vi "探头数据读取.vi"(11 "编号":string) -> ()   [LabVIEW 2016, in "斯坦道多参数.lvlib"]
panel:
  out "运行状态":u16(ring) items=["空闲", "水样测试", "标样核查"]
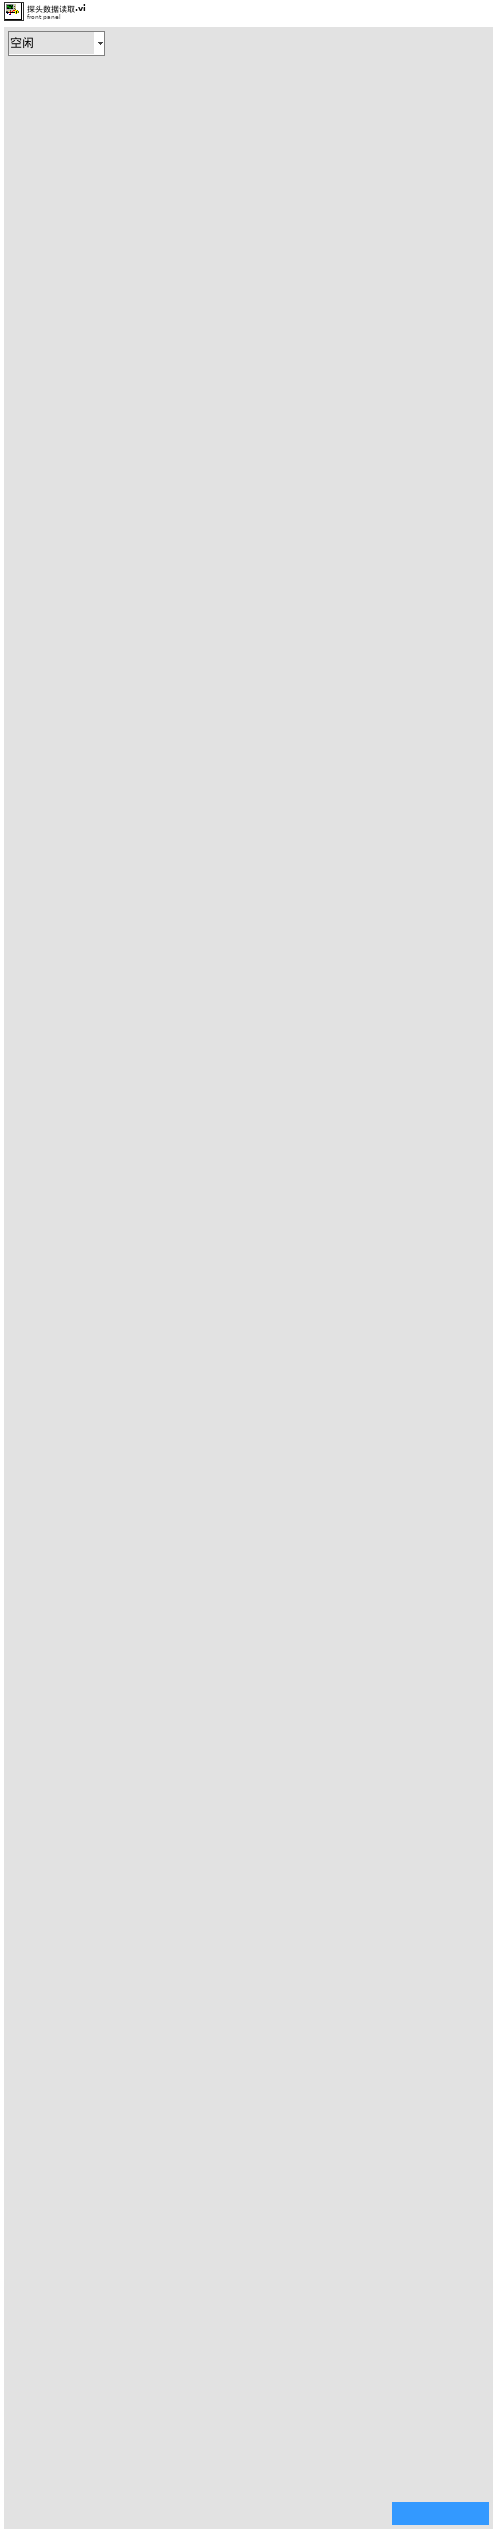
[diagram p1: front panel]
types:
  T1 = enum16{"pH", "DO", "Cond", "Turb", "ORP", "叶绿素a", "藻密度"}
  T2 = cluster{"温度测量值":sgl, "测量值":sgl, "温度偏移修正值":sgl, "信号值":sgl}
  T3 = cluster{"温度测量值":sgl, "DO%":sgl, "DOmg/L":sgl, "温度偏移修正值":sgl}
  T4 = cluster{"CH":u16, "监测值":dbl, "温度偏移修正值":sgl, "信号值":sgl}
  T5 = cluster{"pH探头选择":u16, "DO探头选择":u16, "电导率探头选择":u16, "浊度探头选择":u16, "叶绿素a探头选择":u16, "蓝绿藻探头选择":u16, "orp探头选择":u16}
  T6 = cluster{"电极状态标志":u16, "电极型号标志":u16, "酸碱度测量值":sgl, "温度测量值":sgl, "酸碱度信号值":sgl, "温度信号值":sgl, "酸碱度偏移修正值":sgl, "温度偏移修正值":sgl, "手动温度补偿值":sgl, "酸碱度电极零点":sgl, "酸碱度电极斜率":sgl, "第1点标准值记录":sgl, "第1点信号值记录":sgl, "第1点温度值记录":sgl, "第2点标准值记录":sgl, "第2点信号值记录":sgl, "第2点温度值记录":sgl, "命令滤波设定":u16, "温度模式":enum16{"ATC", "MTC"}, "生产批次":u16, "电极序号":u16, "串口地址":u16, "串口波特率":enum16{"9600", "19200", "115200"}, "串口校验位":enum16{"NONE", "ODD", "EVEN"}, "串口停止位":enum16{"1bit", "2bit"}, "第一点标准值":sgl, "第二点标准值":sgl}
  T7 = cluster{"报警码":u16, "pH数值":sgl, "0X0003_NC":sgl, "温度数据":sgl, "pH原始信号 mv":sgl, "0X0009_NC":string, "产品名称":string, "序列号":string, "硬件版本":string, "软件版本":string, "通讯地址":u16, "波特率":u16, "设备类型":u16, "0X0026_NC":string, "第一点原始数据":sgl, "第一点校准数据":sgl, "第二点原始数据":sgl, "第二点校准数据":sgl, "探头校准命令":u16, "温度校准参数":sgl, "温度校准命令":u16}
  T8 = cluster{"电极状态标志":u16, "电极型号标志":u16, "电导率测量值":sgl, "温度测量值":sgl, "电导率信号值":sgl, "温度信号值":sgl, "温度补偿系数":sgl, "电导率偏移修正值":sgl, "温度偏移修正值":sgl, "手动温度补偿值":sgl, "电导率电极零点":sgl, "电导率电极斜率":sgl, "命令滤波设定":u16, "温度模式":enum16{"ATC", "MTC"}, "生产批次":u16, "电极序号":u16, "串口地址":u16, "串口波特率":enum16{"9600", "19200", "115200"}, "串口校验位":enum16{"NONE", "ODD", "EVEN"}, "串口停止位":enum16{"1bit", "2bit"}, "第一点标准值":sgl, "第二点标准值":sgl}
  T9 = cluster{"报警码":u16, "电导率数据（uS/cm）":sgl, "0x0003 NC":sgl, "温度数据":sgl, "电导率原始信号电阻":sgl, "当前量程":u16, "温度补偿系数":sgl, "0X0009_NC":string, "产品名称":string, "序列号":string, "硬件版本":string, "软件版本":string, "通讯地址":u16, "波特率":u16, "设备类型":u16, "0X0026_NC":string, "第一点原始数据":sgl, "第一点校准数据":sgl, "0X0035_NC":sgl, "0X0037_NC":sgl, "探头校准命令":u16, "温度校准参数":sgl, "温度校准命令":u16}
  T10 = cluster{"电极状态标志":u16, "电极型号标志":u16, "溶解氧测量值":sgl, "温度测量值":sgl, "溶解氧饱和度值":sgl, "盐度补偿值":sgl, "大气压补偿值":sgl, "溶解氧偏移修正值":sgl, "温度偏移修正值":sgl, "手动温度补偿值":sgl, "溶解氧电极零点":sgl, "溶解氧电极斜率":sgl, "第1点标准值记录":sgl, "第1点信号值记录":sgl, "第1点温度值记录":sgl, "第2点标准值记录":sgl, "第2点信号值记录":sgl, "第2点温度值记录":sgl, "命令滤波设定":u16, "温度模式":enum16{"ATC", "MTC"}, "生产批次":u16, "电极序号":u16, "串口地址":u16, "串口波特率":enum16{"9600", "19200", "115200"}, "串口校验位":enum16{"NONE", "ODD", "EVEN"}, "串口停止位":enum16{"1bit", "2bit"}, "第一点标准值":sgl, "第二点标准值":sgl}
  T11 = cluster{"报警码":u16, "溶解氧数值（mg/L）":sgl, "溶解氧数据（%）":sgl, "温度数据":sgl, "溶解氧原始信号 nA":sgl, "大气压力":sgl, "盐度":sgl, "0X0009_NC":string, "产品名称":string, "序列号":string, "硬件版本":string, "软件版本":string, "通讯地址":u16, "波特率":u16, "设备类型":u16, "0X0026_NC":string, "第一点原始数据":sgl, "0X0033 NC":sgl, "第二点原始数据":sgl, "0X0037 NC":sgl, "探头校准命令":u16, "温度校准参数":sgl, "温度校准命令":u16}
  T12 = cluster{"电极状态标志":u16, "电极型号标志":u16, "浊度测量值":sgl, "温度测量值":sgl, "浊度信号值":sgl, "浊度偏移修正值":sgl, "温度偏移修正值":sgl, "手动温度补偿值":sgl, "浊度电极零点":sgl, "浊度电极斜率":sgl, "第1点标准值记录":sgl, "第1点信号值记录":sgl, "第1点温度值记录":sgl, "第2点标准值记录":sgl, "第2点信号值记录":sgl, "第2点温度值记录":sgl, "命令滤波设定":u16, "温度模式":enum16{"ATC", "MTC"}, "生产批次":u16, "电极序号":u16, "串口地址":u16, "串口波特率":enum16{"9600", "19200", "115200"}, "串口校验位":enum16{"NONE", "ODD", "EVEN"}, "串口停止位":enum16{"1bit", "2bit"}, "第一点标准值":sgl, "第二点标准值":sgl, "第三点标准值":sgl}
  T13 = cluster{"报警码":u16, "浊度数值 NTU":sgl, "温度数据":sgl, "原始光强数值":u16, "量程":u16, "平均次数":u16, "清扫模式":u16, "清扫次数":u16, "清扫间隔分钟":u16, "0X000B_NC":string, "产品名称":string, "序列号":string, "硬件版本":string, "软件版本":string, "通讯地址":u16, "波特率":u16, "设备类型":u16, "0X0026_NC":string, "校准量程":u16, "第一点原始光强":u16, "第一点校准数据":sgl, "第二点原始光强":u16, "第二点校准数据":sgl, "第三点原始光强":u16, "第三点校准数据":sgl, "探头校准命令":u16, "温度校准参数":sgl, "温度校准命令":u16}
  T14 = cluster{"电极状态标志":u16, "电极型号标志":u16, "测量值":sgl, "温度测量值":sgl, "信号值":sgl, "温度信号值":sgl, "000AH_NC":sgl, "偏移修正值":sgl, "温度偏移修正值":sgl, "手动温度补偿值":sgl, "命令滤波设定":u16, "温度模式":enum16{"ATC", "MTC"}, "生产批次":u16, "传感器序号":u16, "串口地址":u16, "串口波特率":enum16{"9600", "19200", "115200"}, "串口校验位":enum16{"NONE", "ODD", "EVEN"}, "串口停止位":enum16{"1bit", "2bit"}}
  T15 = cluster{"报警码":u16, "叶绿素a":sgl, "温度数据":sgl, "原始光强数值":u16, "量程":u16, "平均次数":u16, "清扫模式":u16, "清扫次数":u16, "清扫间隔分钟":u16, "0X000B_NC":string, "产品名称":string, "序列号":string, "硬件版本":string, "软件版本":string, "通讯地址":u16, "波特率":u16, "设备类型":u16, "0X0026_NC":string, "校准量程":u16, "第一点原始光强":u16, "第一点校准数据":sgl, "第二点原始光强":u16, "第二点校准数据":sgl, "第三点原始光强":u16, "第三点校准数据":sgl, "探头校准命令":u16, "温度校准参数":sgl, "温度校准命令":u16}
  T16 = cluster{"报警码":u16, "蓝绿藻":sgl, "温度数据":sgl, "原始光强数值":u16, "0X0006_NC":u16, "平均次数":u16, "清扫模式":u16, "清扫次数":u16, "清扫间隔分钟":u16, "0X000B_NC":string, "产品名称":string, "序列号":string, "硬件版本":string, "软件版本":string, "通讯地址":u16, "波特率":u16, "设备类型":u16, "0X0026_NC":string, "0X0030_NC":u16, "第一点原始光强":u16, "第一点校准数据":sgl, "第二点原始光强":u16, "第二点校准数据":sgl, "第三点原始光强":u16, "第三点校准数据":sgl, "探头校准命令":u16, "温度校准参数":sgl, "温度校准命令":u16}
  T17 = enum16{"pH", "DO", "Cond", "Turb", "ORP", "叶绿素a", "藻密度"}[]
  T18 = cluster{"ph":bool, "DO":bool, "Cond":bool, "Turb":bool, "叶绿素a":bool, "藻密度":bool, "ORP":bool}
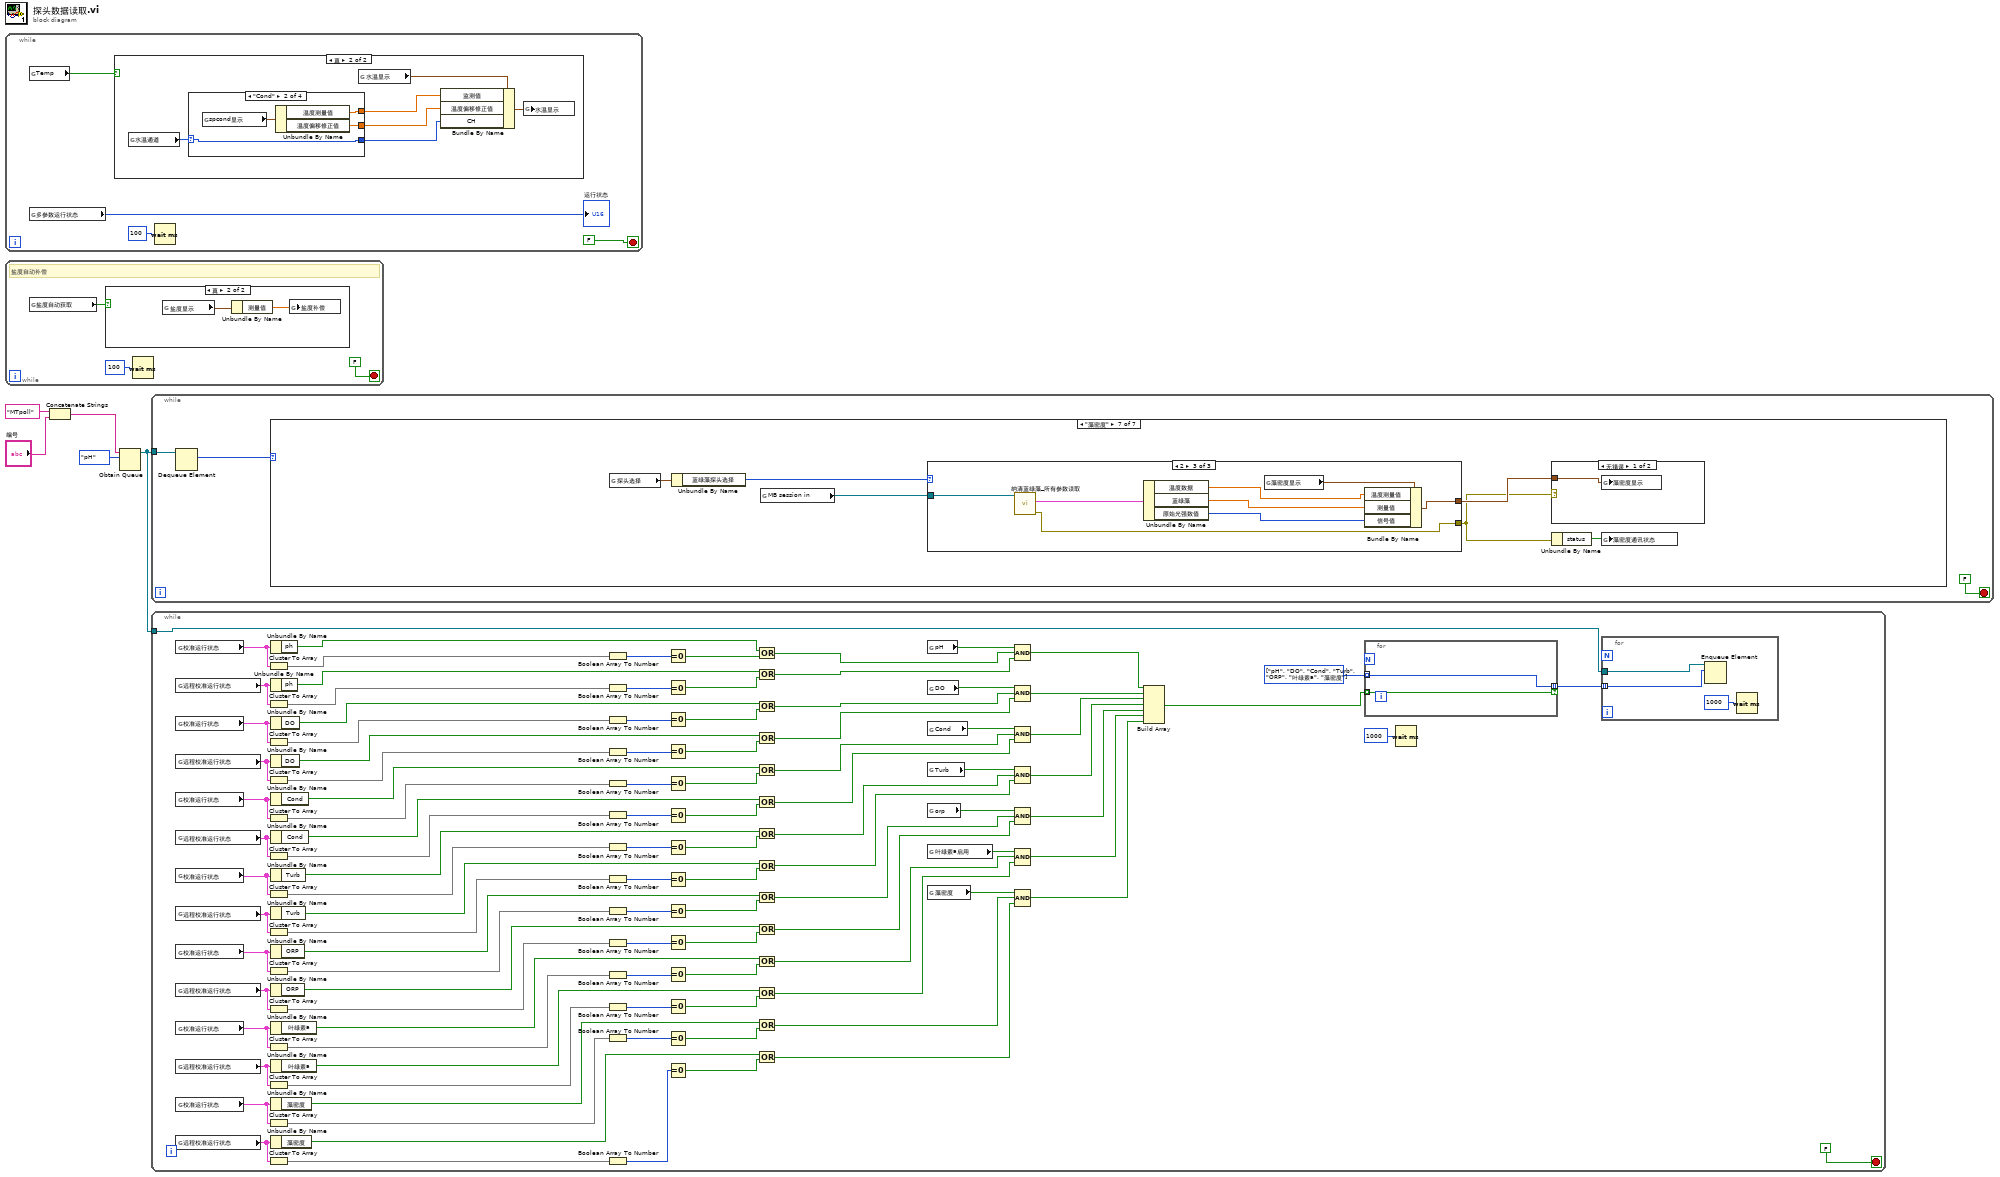
[diagram p0: block diagram]
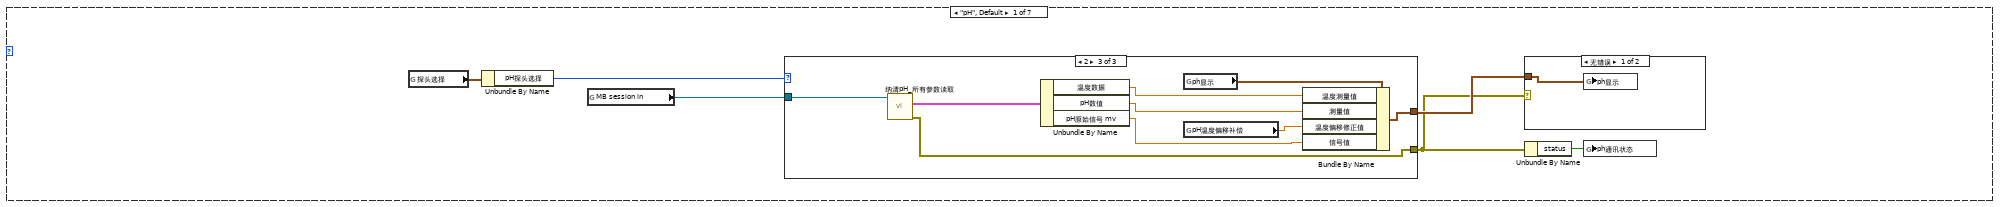
[diagram p2: hidden frame]
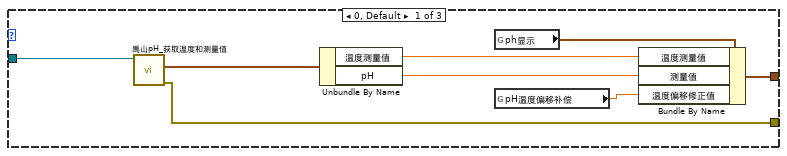
[diagram p3: hidden frame]
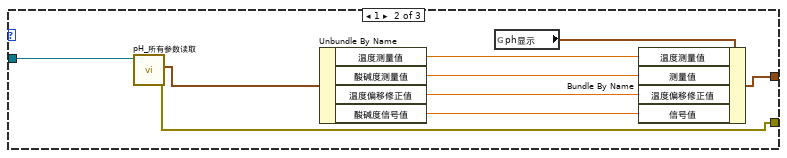
[diagram p4: hidden frame]
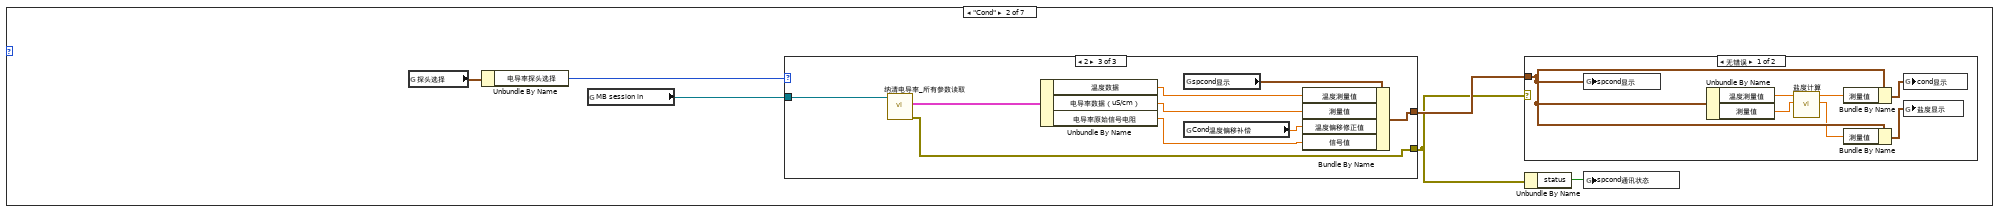
[diagram p6: hidden frame]
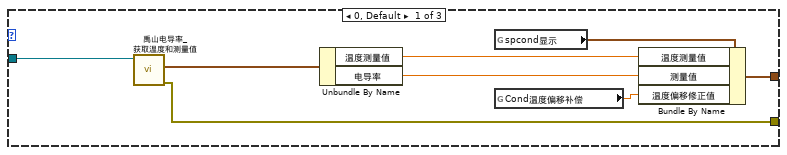
[diagram p7: hidden frame]
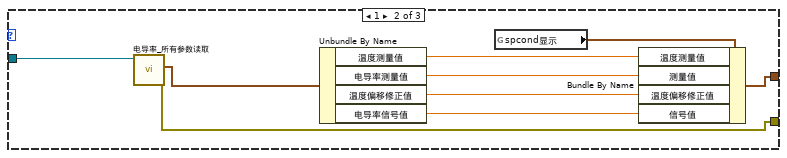
[diagram p8: hidden frame]
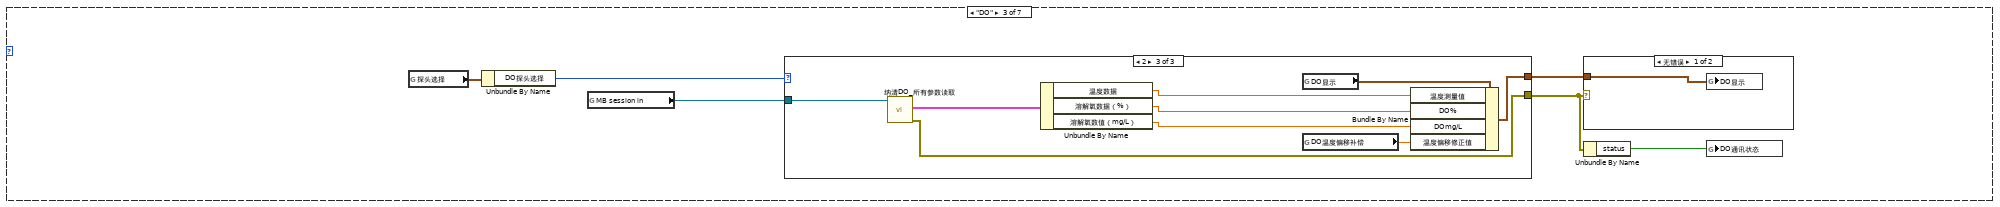
[diagram p10: hidden frame]
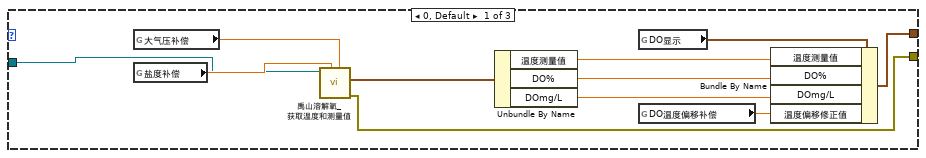
[diagram p11: hidden frame]
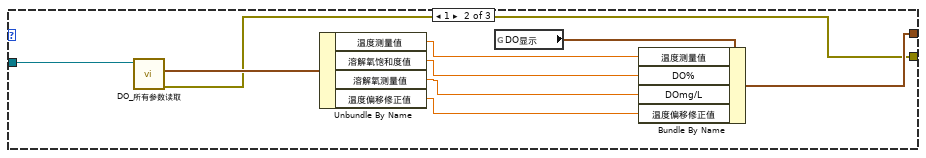
[diagram p12: hidden frame]
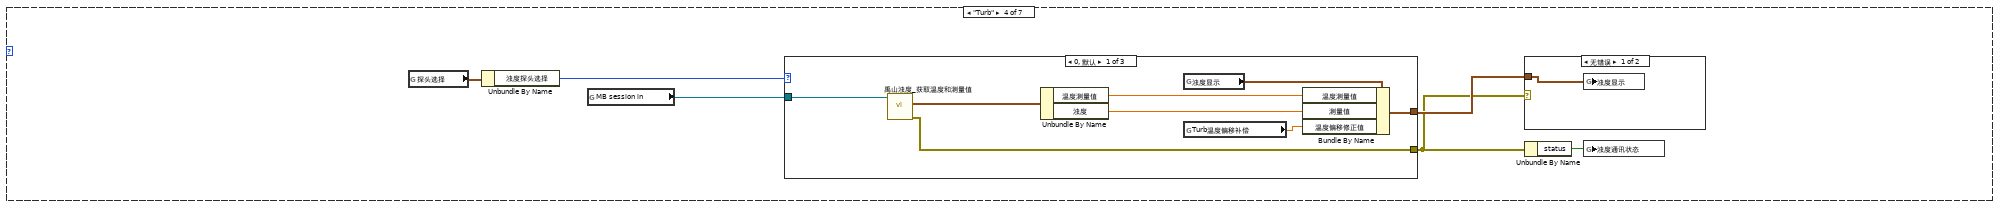
[diagram p14: hidden frame]
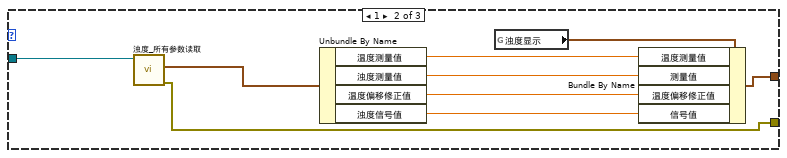
[diagram p15: hidden frame]
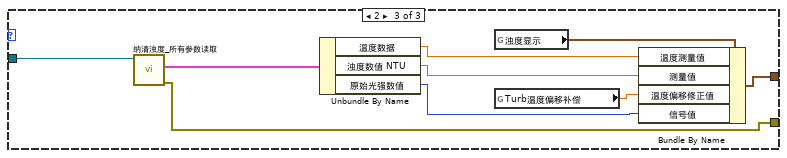
[diagram p16: hidden frame]
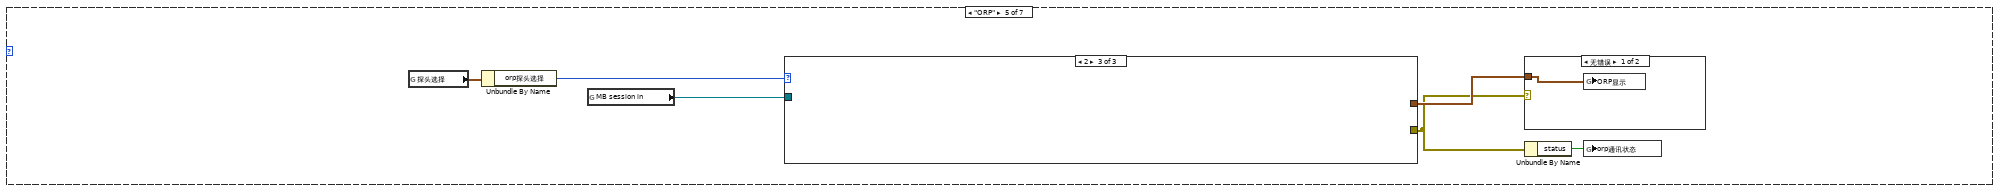
[diagram p18: hidden frame]
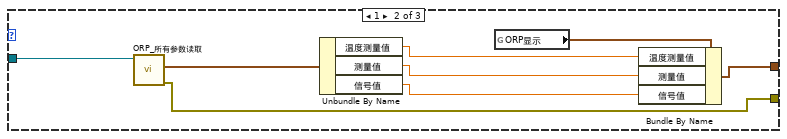
[diagram p20: hidden frame]
diagram:
  n1 = while {
    stop <- FALSE stop-if-true
    n2 = global read "断电保存变量.vi" "Temp"() -> (w7:bool)
    n3 = global read "多参数全局变量.vi" "多参数运行状态"() -> (→"运行状态":u16)
    n4 = case shown="真" w7 {
      frame False {
      }
      frame True {
        n5 = global read "断电保存变量.vi" "水温通道"() -> (w15:enum16{"pH", "Cond", "DO", "Turb"})
        n6 = case shown="\"Cond\"" w15 {
          selector: w15 -> [w19 w23 w27 w31]
          tunnel: [w19 w23 w27 w31] -> w14
          tunnel: [w17 w20 w24 w28] -> w13
          tunnel: [w18 w21 w25 w29] -> w12
          frame "pH", Default {
            n7 = global read "多参数全局变量.vi" "ph显示"() -> (w16:T2)
            n8 = Unbundle By Name(w16) -> ("温度测量值"=w18:sgl, "温度偏移修正值"=w17:sgl)
          }
          frame "Cond" {
            n9 = global read "多参数全局变量.vi" "spcond显示"() -> (w22:T2)
            n10 = Unbundle By Name(w22) -> ("温度测量值"=w21:sgl, "温度偏移修正值"=w20:sgl)
          }
          frame "DO" {
            n11 = global read "多参数全局变量.vi" "DO显示"() -> (w26:T3)
            n12 = Unbundle By Name(w26) -> ("温度测量值"=w25:sgl, "温度偏移修正值"=w24:sgl)
          }
          frame "Turb" {
            n13 = global read "多参数全局变量.vi" "浊度显示"() -> (w30:T2)
            n14 = Unbundle By Name(w30) -> ("温度测量值"=w29:sgl, "温度偏移修正值"=w28:sgl)
          }
        }
        n15 = global read "多参数全局变量.vi" "水温显示"() -> (w10:T4)
        n16 = Bundle By Name(cluster=w10, "监测值"=w12, "温度偏移修正值"=w13, "CH"=w14) -> (w11:T4)
        n17 = global write "多参数全局变量.vi" "水温显示"(w11) -> ()
      }
    }
    n18 = Wait (ms)(milliseconds to wait=u32 100 ("等待时间（毫秒）")) -> ()  [unwired: 1 out]
  }
  n19 = while {
    stop <- FALSE stop-if-true
    # "盐度自动补偿"
    n20 = global read "断电保存变量.vi" "盐度自动获取"() -> (w33:bool)
    n21 = case shown="真" w33 {
      frame False {
      }
      frame True {
        n22 = global read "多参数全局变量.vi" "盐度显示"() -> (w36:T2)
        n23 = Unbundle By Name(w36) -> ("测量值"=w35:sgl)
        n24 = global write "断电保存变量.vi" "盐度补偿"(w35) -> ()
      }
    }
    n25 = Wait (ms)(milliseconds to wait=u32 100 ("等待时间（毫秒）")) -> ()  [unwired: 1 out]
  }
  n26 = Concatenate Strings("MTpoll" ("名称（未命名）"), "编号") -> (w3:string)
  n27 = Obtain Queue(name (unnamed)=w3, element data type=T1."pH" ("枚举")) -> (queue out=w1:refnum<queue>)  [unwired: 3 in, 2 out]
  n28 = while {
    tunnel: w1 -> [w39]
    stop <- FALSE stop-if-true
    n29 = Dequeue Element(queue=w39) -> (element=w38:T1)  [unwired: 2 in, 3 out]
    n30 = case shown="\"藻密度\"" w38 {
      frame "pH", Default {
        n31 = global read "断电保存变量.vi" "探头选择"() -> (w45:T5)
        n32 = Unbundle By Name(w45) -> ("pH探头选择"=w44:u16)
        n33 = global read "多参数全局变量.vi" "MB session in"() -> (w43:refnum<class "MB_Master.lvclass">)
        n34 = case shown="2" w44 {
          tunnel: w43 -> [w53 w62 w69]
          tunnel: [w52 w61 w67] -> w41
          tunnel: [w50 w58 w70] -> w42
          frame 0, Default {
            n35 = call "禹山pH_获取温度和测量值.vi"("MB session in"=w53) -> ("error out"=w52:errorcluster, "输出值"=w49:cluster{"温度测量值":sgl, "ORP":sgl, "pH":sgl})  [unwired: 8 in, 1 out]
            n36 = Unbundle By Name(w49) -> ("温度测量值"=w48:sgl, "pH"=w47:sgl)
            n37 = global read "多参数全局变量.vi" "ph显示"() -> (w51:T2)
            n38 = global read "断电保存变量.vi" "pH温度偏移补偿"() -> (w46:dbl)
            n39 = Bundle By Name(cluster=w51, "温度测量值"=w48, "测量值"=w47, "温度偏移修正值"=w46) -> (w50:T2)
          }
          frame 1 {
            n40 = call "pH_所有参数读取.vi"("MB session in"=w62) -> ("error out"=w61:errorcluster, "输出值"=w60:T6)  [unwired: 8 in, 1 out]
            n41 = Unbundle By Name(w60) -> ("温度测量值"=w55:sgl, "酸碱度测量值"=w56:sgl, "温度偏移修正值"=w57:sgl, "酸碱度信号值"=w54:sgl)
            n42 = global read "多参数全局变量.vi" "ph显示"() -> (w59:T2)
            n43 = Bundle By Name(cluster=w59, "温度测量值"=w55, "测量值"=w56, "温度偏移修正值"=w57, "信号值"=w54) -> (w58:T2)
          }
          frame 2 {
            n44 = call "纳清pH_所有参数读取.vi"("MB session in"=w69) -> ("error out"=w67:errorcluster, "输出值"=w68:T7)  [unwired: 8 in, 1 out]
            n45 = Unbundle By Name(w68) -> ("温度数据"=w66:sgl, "pH数值"=w65:sgl, "pH原始信号 mv"=w63:sgl)
            n46 = global read "多参数全局变量.vi" "ph显示"() -> (w71:T2)
            n47 = global read "断电保存变量.vi" "pH温度偏移补偿"() -> (w64:dbl)
            n48 = Bundle By Name(cluster=w71, "温度测量值"=w66, "测量值"=w65, "温度偏移修正值"=w64, "信号值"=w63) -> (w70:T2)
          }
        }
        n49 = case shown="无错误" w41 {
          tunnel: w42 -> [w72 _]
          frame No Error {
            n50 = global write "多参数全局变量.vi" "ph显示"(w72) -> ()
          }
          frame Error {
          }
        }
        n51 = Unbundle By Name(w41) -> ("status"=w40:bool)
        n52 = global write "多参数全局变量.vi" "ph通讯状态"(w40) -> ()
      }
      frame "Cond" {
        n53 = global read "断电保存变量.vi" "探头选择"() -> (w78:T5)
        n54 = Unbundle By Name(w78) -> ("电导率探头选择"=w77:u16)
        n55 = global read "多参数全局变量.vi" "MB session in"() -> (w75:refnum<class "MB_Master.lvclass">)
        n56 = case shown="2" w77 {
          tunnel: w75 -> [w86 w95 w100]
          tunnel: [w80 w93 w103] -> w76
          tunnel: [w85 w92 w98] -> w74
          frame 0, Default {
            n57 = call "禹山电导率_获取温度和测量值.vi"("MB session in"=w86) -> ("error out"=w85:errorcluster, "输出值"=w83:cluster{"温度测量值":sgl, "电导率":sgl, "错误标志":u16})  [unwired: 8 in, 1 out]
            n58 = Unbundle By Name(w83) -> ("温度测量值"=w82:sgl, "电导率"=w81:sgl)
            n59 = global read "多参数全局变量.vi" "spcond显示"() -> (w84:T2)
            n60 = global read "断电保存变量.vi" "Cond温度偏移补偿"() -> (w79:dbl)
            n61 = Bundle By Name(cluster=w84, "温度测量值"=w82, "测量值"=w81, "温度偏移修正值"=w79) -> (w80:T2)
          }
          frame 1 {
            n62 = call "电导率_所有参数读取.vi"("MB session in"=w95) -> ("error out"=w92:errorcluster, "输出值"=w91:T8)  [unwired: 8 in, 1 out]
            n63 = Unbundle By Name(w91) -> ("温度测量值"=w90:sgl, "电导率测量值"=w89:sgl, "温度偏移修正值"=w88:sgl, "电导率信号值"=w87:sgl)
            n64 = global read "多参数全局变量.vi" "spcond显示"() -> (w94:T2)
            n65 = Bundle By Name(cluster=w94, "温度测量值"=w90, "测量值"=w89, "温度偏移修正值"=w88, "信号值"=w87) -> (w93:T2)
          }
          frame 2 {
            n66 = call "纳清电导率_所有参数读取.vi"("MB session in"=w100) -> ("error out"=w98:errorcluster, "输出值"=w99:T9)  [unwired: 8 in, 1 out]
            n67 = Unbundle By Name(w99) -> ("温度数据"=w102:sgl, "电导率数据（uS/cm）"=w101:sgl, "电导率原始信号电阻"=w96:sgl)
            n68 = global read "多参数全局变量.vi" "spcond显示"() -> (w104:T2)
            n69 = global read "断电保存变量.vi" "Cond温度偏移补偿"() -> (w97:dbl)
            n70 = Bundle By Name(cluster=w104, "温度测量值"=w102, "测量值"=w101, "温度偏移修正值"=w97, "信号值"=w96) -> (w103:T2)
          }
        }
        n71 = case shown="无错误" w74 {
          tunnel: w76 -> [w106 _]
          frame No Error {
            n72 = global write "多参数全局变量.vi" "spcond显示"(w106) -> ()
            n73 = Unbundle By Name(w106) -> ("温度测量值"=w111:sgl, "测量值"=w110:sgl)
            n74 = call "盐度计算.vi"("spCond"=w110, "Temp"=w111) -> ("saltresult"=w105:dbl, "cond"=w109:dbl)  [unwired: 8 in]
            n75 = Bundle By Name(cluster=w106, "测量值"=w109) -> (w108:T2)
            n76 = Bundle By Name(cluster=w106, "测量值"=w105) -> (w107:T2)
            n77 = global write "多参数全局变量.vi" "cond显示"(w108) -> ()
            n78 = global write "多参数全局变量.vi" "盐度显示"(w107) -> ()
          }
          frame Error {
          }
        }
        n79 = Unbundle By Name(w74) -> ("status"=w73:bool)
        n80 = global write "多参数全局变量.vi" "spcond通讯状态"(w73) -> ()
      }
      frame "DO" {
        n81 = global read "断电保存变量.vi" "探头选择"() -> (w117:T5)
        n82 = Unbundle By Name(w117) -> ("DO探头选择"=w116:u16)
        n83 = global read "多参数全局变量.vi" "MB session in"() -> (w114:refnum<class "MB_Master.lvclass">)
        n84 = case shown="2" w116 {
          tunnel: w114 -> [w126 w137 w141]
          tunnel: [w124 w135 w145] -> w115
          tunnel: [w120 w130 w139] -> w113
          frame 0, Default {
            n85 = global read "断电保存变量.vi" "大气压补偿"() -> (w127:dbl)
            n86 = global read "断电保存变量.vi" "盐度补偿"() -> (w128:dbl)
            n87 = call "禹山溶解氧_获取温度和测量值.vi"("大气压补偿"=w127, "盐度补偿"=w128, "MB session in"=w126) -> ("error out"=w120:errorcluster, "输出值"=w118:cluster{"温度测量值":sgl, "DO%":sgl, "DOmg/L":sgl})  [unwired: 6 in, 1 out]
            n88 = Unbundle By Name(w118) -> ("温度测量值"=w123:sgl, "DO%"=w122:sgl, "DOmg/L"=w121:sgl)
            n89 = global read "多参数全局变量.vi" "DO显示"() -> (w125:T3)
            n90 = global read "断电保存变量.vi" "DO温度偏移补偿"() -> (w119:dbl)
            n91 = Bundle By Name(cluster=w125, "温度测量值"=w123, "DO%"=w122, "DOmg/L"=w121, "温度偏移修正值"=w119) -> (w124:T3)
          }
          frame 1 {
            n92 = call "DO_所有参数读取.vi"("MB session in"=w137) -> ("error out"=w130:errorcluster, "输出值"=w134:T10)  [unwired: 8 in, 1 out]
            n93 = Unbundle By Name(w134) -> ("温度测量值"=w131:sgl, "溶解氧饱和度值"=w132:sgl, "溶解氧测量值"=w133:sgl, "温度偏移修正值"=w129:sgl)
            n94 = global read "多参数全局变量.vi" "DO显示"() -> (w136:T3)
            n95 = Bundle By Name(cluster=w136, "温度测量值"=w131, "DO%"=w132, "DOmg/L"=w133, "温度偏移修正值"=w129) -> (w135:T3)
          }
          frame 2 {
            n96 = call "纳清DO_所有参数读取.vi"("MB session in"=w141) -> ("error out"=w139:errorcluster, "输出值"=w140:T11)  [unwired: 8 in, 1 out]
            n97 = Unbundle By Name(w140) -> ("温度数据"=w142:sgl, "溶解氧数据（%）"=w143:sgl, "溶解氧数值（mg/L）"=w144:sgl)
            n98 = global read "多参数全局变量.vi" "DO显示"() -> (w146:T3)
            n99 = global read "断电保存变量.vi" "DO温度偏移补偿"() -> (w138:dbl)
            n100 = Bundle By Name(cluster=w146, "温度测量值"=w142, "DO%"=w143, "DOmg/L"=w144, "温度偏移修正值"=w138) -> (w145:T3)
          }
        }
        n101 = case shown="无错误" w113 {
          tunnel: w115 -> [w147 _]
          frame No Error {
            n102 = global write "多参数全局变量.vi" "DO显示"(w147) -> ()
          }
          frame Error {
          }
        }
        n103 = Unbundle By Name(w113) -> ("status"=w112:bool)
        n104 = global write "多参数全局变量.vi" "DO通讯状态"(w112) -> ()
      }
      frame "Turb" {
        n105 = global read "断电保存变量.vi" "探头选择"() -> (w153:T5)
        n106 = Unbundle By Name(w153) -> ("浊度探头选择"=w152:u16)
        n107 = global read "多参数全局变量.vi" "MB session in"() -> (w150:refnum<class "MB_Master.lvclass">)
        n108 = case shown="0, 默认" w152 {
          tunnel: w150 -> [w161 w170 w175]
          tunnel: [w159 w165 w176] -> w151
          tunnel: [w158 w164 w174] -> w149
          frame 0, Default {
            n109 = call "禹山浊度_获取温度和测量值.vi"("MB session in"=w161) -> ("error out"=w158:errorcluster, "输出值"=w157:cluster{"温度测量值":sgl, "浊度":sgl})  [unwired: 8 in, 1 out]
            n110 = Unbundle By Name(w157) -> ("温度测量值"=w156:sgl, "浊度"=w155:sgl)
            n111 = global read "多参数全局变量.vi" "浊度显示"() -> (w160:T2)
            n112 = global read "断电保存变量.vi" "Turb温度偏移补偿"() -> (w154:dbl)
            n113 = Bundle By Name(cluster=w160, "温度测量值"=w156, "测量值"=w155, "温度偏移修正值"=w154) -> (w159:T2)
          }
          frame 1 {
            n114 = call "浊度_所有参数读取.vi"("MB session in"=w170) -> ("error out"=w164:errorcluster, "输出值"=w169:T12)  [unwired: 8 in, 1 out]
            n115 = Unbundle By Name(w169) -> ("温度测量值"=w167:sgl, "浊度测量值"=w166:sgl, "温度偏移修正值"=w163:sgl, "浊度信号值"=w162:sgl)
            n116 = global read "多参数全局变量.vi" "浊度显示"() -> (w168:T2)
            n117 = Bundle By Name(cluster=w168, "温度测量值"=w167, "测量值"=w166, "温度偏移修正值"=w163, "信号值"=w162) -> (w165:T2)
          }
          frame 2 {
            n118 = call "纳清浊度_所有参数读取.vi"("MB session in"=w175) -> ("error out"=w174:errorcluster, "输出值"=w173:T13)  [unwired: 8 in, 1 out]
            n119 = Unbundle By Name(w173) -> ("温度数据"=w178:sgl, "浊度数值 NTU"=w177:sgl, "原始光强数值"=w171:u16)
            n120 = global read "多参数全局变量.vi" "浊度显示"() -> (w179:T2)
            n121 = global read "断电保存变量.vi" "Turb温度偏移补偿"() -> (w172:dbl)
            n122 = Bundle By Name(cluster=w179, "温度测量值"=w178, "测量值"=w177, "温度偏移修正值"=w172, "信号值"=w171) -> (w176:T2)
          }
        }
        n123 = case shown="无错误" w149 {
          tunnel: w151 -> [w180 _]
          frame No Error {
            n124 = global write "多参数全局变量.vi" "浊度显示"(w180) -> ()
          }
          frame Error {
          }
        }
        n125 = Unbundle By Name(w149) -> ("status"=w148:bool)
        n126 = global write "多参数全局变量.vi" "浊度通讯状态"(w148) -> ()
      }
      frame "ORP" {
        n127 = global read "断电保存变量.vi" "探头选择"() -> (w185:T5)
        n128 = Unbundle By Name(w185) -> ("orp探头选择"=w184:u16)
        n129 = global read "多参数全局变量.vi" "MB session in"() -> (w183:refnum<class "MB_Master.lvclass">)
        n130 = case shown="2" w184 {
          tunnel: [_ w189 _] -> w182
          tunnel: w183 -> [_ w194 _]
          tunnel: [_ w187 _] -> w186
          frame 0, Default {
          }
          frame 1 {
            n131 = call "ORP_所有参数读取.vi"("MB session in"=w194) -> ("error out"=w189:errorcluster, "输出值"=w191:T14)  [unwired: 8 in, 1 out]
            n132 = Unbundle By Name(w191) -> ("温度测量值"=w192:sgl, "测量值"=w193:sgl, "信号值"=w188:sgl)
            n133 = global read "多参数全局变量.vi" "ORP显示"() -> (w190:T2)
            n134 = Bundle By Name(cluster=w190, "温度测量值"=w192, "测量值"=w193, "信号值"=w188) -> (w187:T2)
          }
          frame 2 {
          }
        }
        n135 = case shown="无错误" w182 {
          tunnel: w186 -> [w195 _]
          frame No Error {
            n136 = global write "多参数全局变量.vi" "ORP显示"(w195) -> ()
          }
          frame Error {
          }
        }
        n137 = Unbundle By Name(w182) -> ("status"=w181:bool)
        n138 = global write "多参数全局变量.vi" "orp通讯状态"(w181) -> ()
      }
      frame "叶绿素a" {
        n139 = global read "断电保存变量.vi" "探头选择"() -> (w200:T5)
        n140 = Unbundle By Name(w200) -> ("叶绿素a探头选择"=w199:u16)
        n141 = global read "多参数全局变量.vi" "MB session in"() -> (w198:refnum<class "MB_Master.lvclass">)
        n142 = case shown="2" w199 {
          tunnel: [w208 _ w214] -> w197
          tunnel: w198 -> [w207 _ w216]
          tunnel: [w205 _ w213] -> w201
          frame 0, Default {
            n143 = call "叶绿素a_获取温度和叶绿素值.vi"("MB session in"=w207) -> ("error out"=w208:errorcluster, "输出值"=w204:cluster{"温度测量值":sgl, "叶绿素测量值":sgl, "错误标志":u16})  [unwired: 8 in, 1 out]
            n144 = Unbundle By Name(w204) -> ("温度测量值"=w202:sgl, "叶绿素测量值"=w203:sgl)
            n145 = global read "多参数全局变量.vi" "叶绿素a显示"() -> (w206:T2)
            n146 = Bundle By Name(cluster=w206, "温度测量值"=w202, "测量值"=w203) -> (w205:T2)
          }
          frame 1 {
          }
          frame 2 {
            n147 = call "纳清叶绿素a_所有参数读取.vi"("MB session in"=w216) -> ("error out"=w214:errorcluster, "输出值"=w212:T15)  [unwired: 8 in, 1 out]
            n148 = Unbundle By Name(w212) -> ("温度数据"=w210:sgl, "叶绿素a"=w211:sgl, "原始光强数值"=w209:u16)
            n149 = global read "多参数全局变量.vi" "叶绿素a显示"() -> (w215:T2)
            n150 = Bundle By Name(cluster=w215, "温度测量值"=w210, "测量值"=w211, "信号值"=w209) -> (w213:T2)
          }
        }
        n151 = case shown="无错误" w197 {
          tunnel: w201 -> [w217 _]
          frame No Error {
            n152 = global write "多参数全局变量.vi" "叶绿素a显示"(w217) -> ()
          }
          frame Error {
          }
        }
        n153 = Unbundle By Name(w197) -> ("status"=w196:bool)
        n154 = global write "多参数全局变量.vi" "叶绿素a通讯状态"(w196) -> ()
      }
      frame "藻密度" {
        n155 = global read "断电保存变量.vi" "探头选择"() -> (w222:T5)
        n156 = Unbundle By Name(w222) -> ("蓝绿藻探头选择"=w221:u16)
        n157 = global read "多参数全局变量.vi" "MB session in"() -> (w220:refnum<class "MB_Master.lvclass">)
        n158 = case shown="2" w221 {
          tunnel: [_ _ w229] -> w219
          tunnel: w220 -> [_ _ w231]
          tunnel: [_ _ w228] -> w223
          frame 0, Default {
          }
          frame 1 {
          }
          frame 2 {
            n159 = call "纳清蓝绿藻_所有参数读取.vi"("MB session in"=w231) -> ("error out"=w229:errorcluster, "输出值"=w227:T16)  [unwired: 8 in, 1 out]
            n160 = Unbundle By Name(w227) -> ("温度数据"=w226:sgl, "蓝绿藻"=w225:sgl, "原始光强数值"=w224:u16)
            n161 = global read "多参数全局变量.vi" "藻密度显示"() -> (w230:T2)
            n162 = Bundle By Name(cluster=w230, "温度测量值"=w226, "测量值"=w225, "信号值"=w224) -> (w228:T2)
          }
        }
        n163 = case shown="无错误" w219 {
          tunnel: w223 -> [w232 _]
          frame No Error {
            n164 = global write "多参数全局变量.vi" "藻密度显示"(w232) -> ()
          }
          frame Error {
          }
        }
        n165 = Unbundle By Name(w219) -> ("status"=w218:bool)
        n166 = global write "多参数全局变量.vi" "藻密度通讯状态"(w218) -> ()
      }
    }
  }
  n167 = while {
    tunnel: w1 -> [w336]
    stop <- FALSE stop-if-true
    w235 = T17 [enum."pH", enum."DO", enum."Cond", enum."Turb", enum."ORP", enum."叶绿素a", enum."藻密度"] items=["pH", "DO", "Cond", "Turb", "ORP", "叶绿素a", "藻密度"]
    n168 = global read "多参数全局变量.vi" "校准运行状态"() -> (w322:T18)
    n169 = global read "多参数全局变量.vi" "远程校准运行状态"() -> (w333:T18)
    n170 = global read "多参数全局变量.vi" "校准运行状态"() -> (w296:T18)
    n171 = global read "多参数全局变量.vi" "远程校准运行状态"() -> (w307:T18)
    n172 = global read "多参数全局变量.vi" "校准运行状态"() -> (w321:T18)
    n173 = global read "多参数全局变量.vi" "远程校准运行状态"() -> (w310:T18)
    n174 = global read "多参数全局变量.vi" "校准运行状态"() -> (w283:T18)
    n175 = global read "多参数全局变量.vi" "远程校准运行状态"() -> (w294:T18)
    n176 = global read "多参数全局变量.vi" "校准运行状态"() -> (w270:T18)
    n177 = global read "多参数全局变量.vi" "远程校准运行状态"() -> (w281:T18)
    n178 = global read "多参数全局变量.vi" "校准运行状态"() -> (w269:T18)
    n179 = global read "多参数全局变量.vi" "远程校准运行状态"() -> (w258:T18)
    n180 = global read "多参数全局变量.vi" "校准运行状态"() -> (w244:T18)
    n181 = global read "多参数全局变量.vi" "远程校准运行状态"() -> (w255:T18)
    n182 = Cluster To Array(cluster=w322) -> (array=w327:bool[])
    n183 = Cluster To Array(cluster=w333) -> (array=w329:bool[])
    n184 = Cluster To Array(cluster=w296) -> (array=w301:bool[])
    n185 = Cluster To Array(cluster=w307) -> (array=w303:bool[])
    n186 = Cluster To Array(cluster=w321) -> (array=w316:bool[])
    n187 = Cluster To Array(cluster=w310) -> (array=w314:bool[])
    n188 = Cluster To Array(cluster=w283) -> (array=w288:bool[])
    n189 = Cluster To Array(cluster=w294) -> (array=w290:bool[])
    n190 = Cluster To Array(cluster=w270) -> (array=w275:bool[])
    n191 = Cluster To Array(cluster=w281) -> (array=w277:bool[])
    n192 = Cluster To Array(cluster=w269) -> (array=w264:bool[])
    n193 = Cluster To Array(cluster=w258) -> (array=w262:bool[])
    n194 = Cluster To Array(cluster=w244) -> (array=w249:bool[])
    n195 = Cluster To Array(cluster=w255) -> (array=w251:bool[])
    n196 = Unbundle By Name(w322) -> ("ph"=w324:bool)
    n197 = Unbundle By Name(w333) -> ("ph"=w332:bool)
    n198 = Unbundle By Name(w296) -> ("DO"=w298:bool)
    n199 = Unbundle By Name(w307) -> ("DO"=w306:bool)
    n200 = Unbundle By Name(w321) -> ("Cond"=w319:bool)
    n201 = Unbundle By Name(w310) -> ("Cond"=w311:bool)
    n202 = Unbundle By Name(w283) -> ("Turb"=w285:bool)
    n203 = Unbundle By Name(w294) -> ("Turb"=w293:bool)
    n204 = Unbundle By Name(w270) -> ("ORP"=w272:bool)
    n205 = Unbundle By Name(w281) -> ("ORP"=w280:bool)
    n206 = Unbundle By Name(w269) -> ("叶绿素a"=w267:bool)
    n207 = Unbundle By Name(w258) -> ("叶绿素a"=w259:bool)
    n208 = Unbundle By Name(w244) -> ("藻密度"=w246:bool)
    n209 = Unbundle By Name(w255) -> ("藻密度"=w254:bool)
    n210 = Boolean Array To Number(Boolean array=w327) -> (number=w326:u32)
    n211 = Boolean Array To Number(Boolean array=w329) -> (number=w330:u32)
    n212 = Boolean Array To Number(Boolean array=w301) -> (number=w300:u32)
    n213 = Boolean Array To Number(Boolean array=w303) -> (number=w304:u32)
    n214 = Boolean Array To Number(Boolean array=w316) -> (number=w317:u32)
    n215 = Boolean Array To Number(Boolean array=w314) -> (number=w313:u32)
    n216 = Boolean Array To Number(Boolean array=w288) -> (number=w287:u32)
    n217 = Boolean Array To Number(Boolean array=w290) -> (number=w291:u32)
    n218 = Boolean Array To Number(Boolean array=w275) -> (number=w274:u32)
    n219 = Boolean Array To Number(Boolean array=w277) -> (number=w278:u32)
    n220 = Boolean Array To Number(Boolean array=w264) -> (number=w265:u32)
    n221 = Boolean Array To Number(Boolean array=w262) -> (number=w261:u32)
    n222 = Boolean Array To Number(Boolean array=w249) -> (number=w248:u32)
    n223 = Boolean Array To Number(Boolean array=w251) -> (number=w252:u32)
    n224 = Equal To 0?(x=w326) -> (x = 0?=w325:bool)
    n225 = Equal To 0?(x=w330) -> (x = 0?=w331:bool)
    n226 = Equal To 0?(x=w300) -> (x = 0?=w299:bool)
    n227 = Equal To 0?(x=w304) -> (x = 0?=w305:bool)
    n228 = Equal To 0?(x=w317) -> (x = 0?=w318:bool)
    n229 = Equal To 0?(x=w313) -> (x = 0?=w312:bool)
    n230 = Equal To 0?(x=w287) -> (x = 0?=w286:bool)
    n231 = Equal To 0?(x=w291) -> (x = 0?=w292:bool)
    n232 = Equal To 0?(x=w274) -> (x = 0?=w273:bool)
    n233 = Equal To 0?(x=w278) -> (x = 0?=w279:bool)
    n234 = Equal To 0?(x=w265) -> (x = 0?=w266:bool)
    n235 = Equal To 0?(x=w261) -> (x = 0?=w260:bool)
    n236 = Equal To 0?(x=w248) -> (x = 0?=w247:bool)
    n237 = Equal To 0?(x=w252) -> (x = 0?=w253:bool)
    n238 = Or(x=w324, y=w325) -> (x .or. y?=w323:bool)
    n239 = Or(x=w332, y=w331) -> (x .or. y?=w334:bool)
    n240 = Or(x=w298, y=w299) -> (x .or. y?=w297:bool)
    n241 = Or(x=w306, y=w305) -> (x .or. y?=w308:bool)
    n242 = Or(x=w319, y=w318) -> (x .or. y?=w320:bool)
    n243 = Or(x=w311, y=w312) -> (x .or. y?=w309:bool)
    n244 = Or(x=w285, y=w286) -> (x .or. y?=w284:bool)
    n245 = Or(x=w293, y=w292) -> (x .or. y?=w295:bool)
    n246 = Or(x=w272, y=w273) -> (x .or. y?=w271:bool)
    n247 = Or(x=w280, y=w279) -> (x .or. y?=w282:bool)
    n248 = Or(x=w267, y=w266) -> (x .or. y?=w268:bool)
    n249 = Or(x=w259, y=w260) -> (x .or. y?=w257:bool)
    n250 = Or(x=w246, y=w247) -> (x .or. y?=w245:bool)
    n251 = Or(x=w254, y=w253) -> (x .or. y?=w256:bool)
    n252 = global read "断电保存变量.vi" "pH"() -> (w328:bool)
    n253 = global read "断电保存变量.vi" "DO"() -> (w302:bool)
    n254 = global read "断电保存变量.vi" "Cond"() -> (w315:bool)
    n255 = global read "断电保存变量.vi" "Turb"() -> (w289:bool)
    n256 = global read "断电保存变量.vi" "orp"() -> (w276:bool)
    n257 = global read "断电保存变量.vi" "叶绿素a启用"() -> (w263:bool)
    n258 = global read "断电保存变量.vi" "藻密度"() -> (w250:bool)
    n259 = Compound Arithmetic op=AND ("复合运算")(w328, w323, w334) -> (w243:bool)
    n260 = Compound Arithmetic op=AND ("复合运算")(w302, w297, w308) -> (w242:bool)
    n261 = Compound Arithmetic op=AND ("复合运算")(w315, w320, w309) -> (w241:bool)
    n262 = Compound Arithmetic op=AND ("复合运算")(w289, w284, w295) -> (w240:bool)
    n263 = Compound Arithmetic op=AND ("复合运算")(w276, w271, w282) -> (w239:bool)
    n264 = Compound Arithmetic op=AND ("复合运算")(w263, w268, w257) -> (w238:bool)
    n265 = Compound Arithmetic op=AND ("复合运算")(w250, w245, w256) -> (w237:bool)
    n266 = Build Array(w243, w242, w241, w240, w239, w238, w237) -> (w236:bool[])
    n267 = for {
      tunnel: w236 -> [w340] mode=indexing
      tunnel: w235 -> [w341] mode=indexing
      tunnel: [w341] -> w234 mode=indexing if=w340
    }
    n268 = Wait (ms)(milliseconds to wait=u32 1000 ("等待时间（毫秒）")) -> ()  [unwired: 1 out]
    n269 = for {
      tunnel: w336 -> [w339]
      tunnel: w234 -> [w338] mode=indexing
      n270 = Enqueue Element(queue=w339, element=w338) -> ()  [unwired: 2 in, 3 out]
      n271 = Wait (ms)(milliseconds to wait=u32 1000 ("等待时间（毫秒）")) -> ()  [unwired: 1 out]
    }
  }
